vi "New.vi"(8 "Error In":errorcluster, 11 "Key":string) -> (0 "Error Out":errorcluster, 3 "End Section":refnum<class "EndSection.lvclass">)   [LabVIEW 2017, in "Mustache.lvlib" / "Tokens.lvlib" / "EndSection.lvclass"]
uses:
  EndSection.lvclass
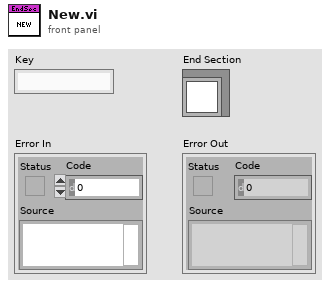
[diagram p1: front panel]
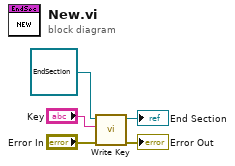
[diagram p0: block diagram]
diagram:
  n1 = call-dynamic "Write Key.vi"("Error In"="Error In", "Key"="Key", "Variable In"=refnum<class "EndSection.lvclass"> refnum ("Mustache.lvlib:Tokens.lvlib:EndSection.lvclass")) -> ("Error Out"=→"Error Out":errorcluster, "Variable Out"=→"End Section":refnum<class "EndSection.lvclass">)  [unwired: 7 in]
